vi "Alazar module.vi"(7 "FFT Channel":u32(ring)=1 items=["A"=1, "B"=2, "A + B"=3, "C"=4, "A + C"=5, "A + B"=6, "D"=8, "A + D"=9, "B + D"=10, "C + D"=12, "A + B + C + D"=15], 8 "Error in":errorcluster, 10 "Scan Status in":T1) -> (0 "Error Out":errorcluster, 3 "FFT Buffer":sgl[](array[numeric]))   [LabVIEW 2018]
uses:
  Controls/scan status.ctl
  Hardware Mfg/AlazarTech SDK/Controls/Alazar Engine Actions.ctl
  Controls/FGV Actions.ctl
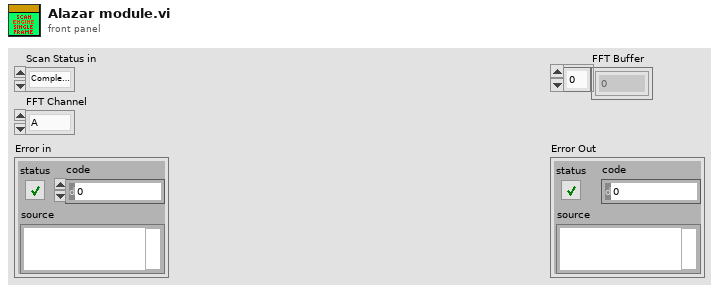
[diagram p1: front panel]
types:
  T1 = typedef "scan status.ctl" = enum16{"Complete Scan", "Start", "Continue Scan", "Finish Scan"}
  T2 = typedef "Alazar Engine Actions.ctl" = enum16{"Init", "Config Clock", "Config Ch", "Config Trig", "Config Non-FFT Acq.", "Non-FFT Acquire", "start acquire", "Config Acq.", "Acquire", "UnInit"}
  T3 = typedef "FGV Actions.ctl" = enum16{"Init", "Set", "Get", "Clear"}
  T4 = enum16{"Configure channels", "Write Scan Pattern", "Start Galvo Task", "Is Task Done?", "Stop Galvo", "Uninit", "Init: Calc scan pattern"}
  T5 = typedef "System Parameters.ctl" = cluster{"Optical Parameters":T6, "Vibratome":T7, "Table Stages":T8, "Imaging Parameter":T11, "Galvo HW Parameters":cluster{"Analog Out Channel":tag, "Min Voltage":dbl, "Max Voltage":dbl, "Pixel Clock Source":tag, "Sample Rate":dbl, "Line Clock Out Ch":tag}, "Alazar parameters":T13, "Mosaic Paramter":cluster{"X Axis":cluster{"Start [mm]":dbl, "Steps [pts]":u16, "End [mm]":dbl}, "Y Axis":cluster{"Start [mm]":dbl, "Steps [pts]":u16, "End [mm]":dbl}, "Scan Pattern":enum16{"Uni-directional", "Bi-Directional", "Spiral Out", "Spiral In"}, "Overlap Options":cluster{"Overlap Type":enum16{"No Overlap", "X Only", "Y Only", "X and Y"}, "Percent Overlap":u8, "Justify":enum16{"Start", "Center", "End"}}}, "Vibratome Axis":cluster{"Start [mm](next cut height)":dbl, "thick[um]":dbl, "#slices":dbl}}
  T6 = typedef "Optical Parameters.ctl" = cluster{"Obj. Focal Length [mm]":dbl, "Scan Lens EFL[mm]":dbl, "Tube Lens EFL[mm]":dbl, "Galvo V Range (+/-)":dbl, "Galvo Max Half Angle [Deg]":dbl, "Max Galvo Range[%]":dbl}
  T7 = typedef "Vibratome Parameters.ctl" = cluster{"Z Bottom [mm]":dbl, "Pre Cut Dwell [s]":dbl, "Blade Frequency [RPM]":u16, "Slice Speed [mm/s]":dbl, "Post Cut Dwell [s]":dbl, "Ramp Time [s]":dbl, "Start X [mm]":dbl, "Start Y [mm]":dbl, "Slice Length [mm]":dbl, "Slice Axis":enum16{"X Axis", "Y Axis", "Z Axis"}, "Controller VISA Ref":refnum<visa-resource-name>}
  T8 = typedef "Translation Stage Parameters.ctl" = cluster{"X Stage":T9, "Y Stage":T9, "Z Stage":T9}
  T9 = typedef "Translation Stage Cluster.ctl" = cluster{"Position":dbl, "Is.Enabled?":bool, "Is.Connected?":bool, "Device SN":string, "AccelerationMaximum":dbl, "VelocityMaximum":dbl, "Acceleration":dbl, "Velocity":dbl, "waitTimeout (ms)":i32, "Model":T10, "Is.Homed?":bool}
  T10 = typedef "Translation Stage Types.ctl" = enum16{"None", "Thorlabs LTS", "Thorlabs MLJ"}
  T11 = typedef "Imaging Parameters.ctl" = cluster{"Raster Scan Direction":T12, "Pixel Dwell Time [Clock Cycles]":u16, "Flyback Time [Clock Cycles]":u16, "XY Center [um]":cluster{"X":dbl, "Y":dbl}, "Pixel Step Size [um]":dbl, "XY Image Size":enum16{"32 x 32", "64 x 64", "128 x 128", "256 x 256", "512 x 512", "1024 x 1024", "2048 x 2048"}, "Custom":bool, "Custom Size":cluster{"X":u16, "Y":u16}, "Line Averages":u8}
  T12 = typedef "Scan Direction.ctl" = enum16{"Uni Directional", "Bi Directional", "None"}
  T13 = typedef "Alazar parameters.ctl" = cluster{"Trigger Settings":cluster{"General Trigger Settings":T14, "Trigger Engine 1":T15, "Trigger Engine 2":T15}, "Capture Clock":T16, "Device ID":T17, "Ch A Input Control":T18, "Ch B Input Control":T18, "Acq Settings":T19}
  T14 = typedef "General Trigger Settings.ctl" = cluster{"Trigger Operation":u32, "Coupling ID":u32, "Range ID":u32, "Delay":u32, "Timeout Ticks":u32, "Mode":u32, "Parameter":u32}
  T15 = typedef "Trigger Engine Controls.ctl" = cluster{"Trigger Engine":u32, "Source":u32, "Slope":u32, "Level":u32}
  T16 = typedef "Clock Controls.ctl" = cluster{"Sample Rate":u32, "Decimation":u32, "Source":u32, "Edge":u32}
  T17 = typedef "Alazar Device ID.ctl" = cluster{"System ID":u32, "Board ID":u32}
  T18 = typedef "Channel Input Controls.ctl" = cluster{"Channel":u8, "Coupling":u32, "Range":u32, "Impedance":u32}
  T19 = typedef "Alazar Acquisition Settings.ctl" = cluster{"Record Length":u32, "Offset":u32, "Records Per Buffer":u32, "Records Count (Records/Acq)":u32, "Window Type":u32, "Footer":u32, "Samples per record":u32, "Output Format":u32}
  T20 = cluster{"General Trigger Settings":T14, "Trigger Engine 1":T15, "Trigger Engine 2":T15}
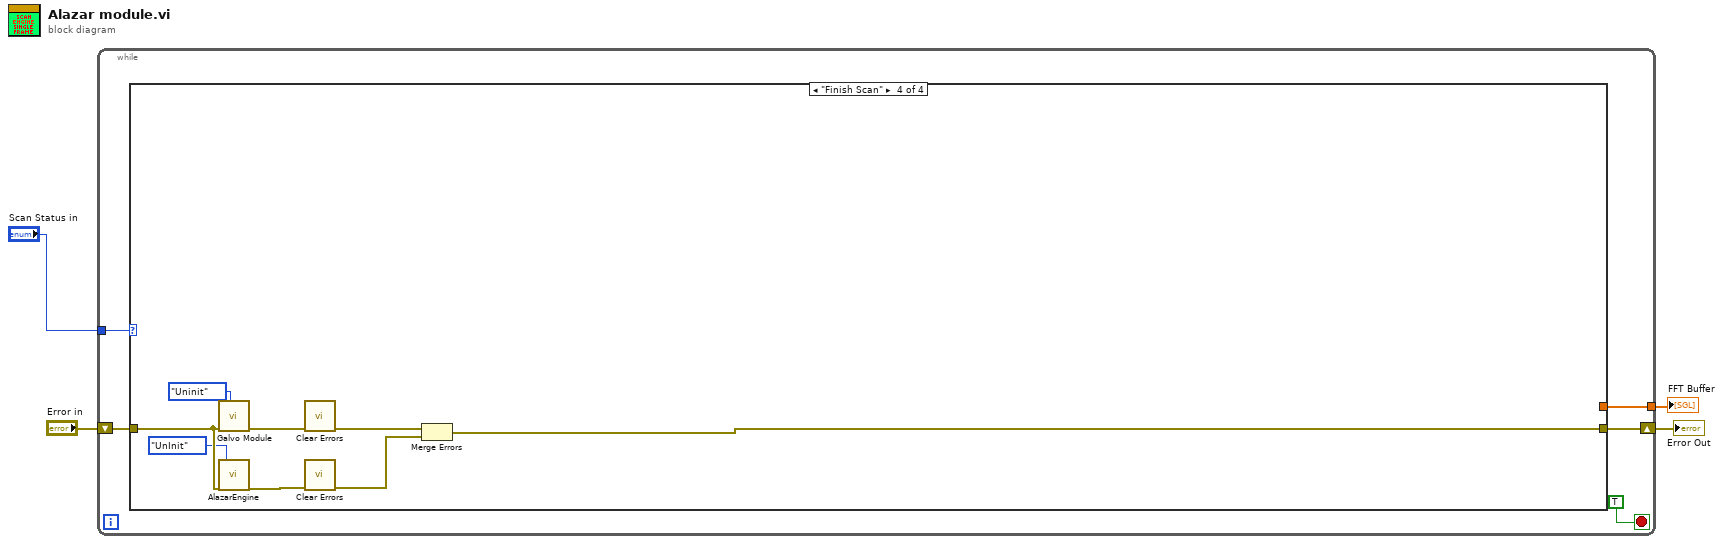
[diagram p0: block diagram]
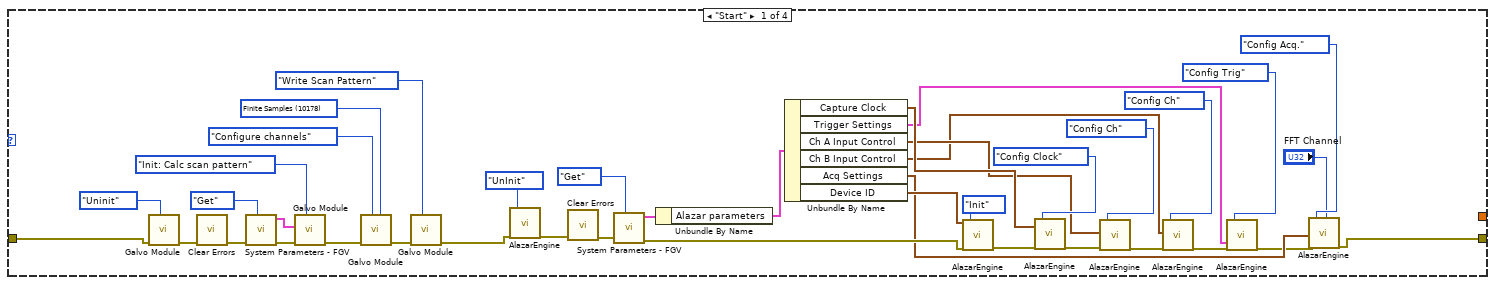
[diagram p2: hidden frame]
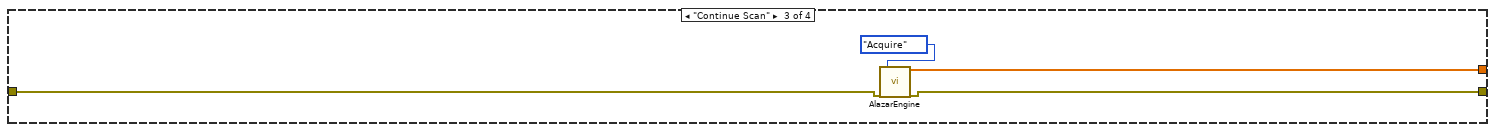
[diagram p4: hidden frame]
diagram:
  n1 = while {
    shift-right: [w8] -> w3
    shift-left: "Error in" -> [w6]
    tunnel: "Scan Status in" -> [w7]
    tunnel: [w5] -> w1
    stop <- TRUE ("Status In") stop-if-true
    n2 = case shown="\"Finish Scan\"" w7 {
      tunnel: w6 -> [w37 w50 w53 w59]
      tunnel: [w11 w50 w52 w56] -> w8
      tunnel: [_ _ w51 _] -> w5
      frame "Start" {
        w46 = 10178 items=["Finite Samples"=10178, "Continuous Samples"=10123, "Hardware Timed Single Point"=12522] ("sample mode")
        n3 = call "Galvo Module.vi"("Action"=T4."Uninit", "error in (no error)"=w37) -> ("error out"=w40:errorcluster)  [unwired: 8 in, 1 out]
        n4 = call <vilib>:"Clear Errors.vi"("error in (no error)"=w40) -> ("error out"=w38:errorcluster)  [unwired: 5 in, 1 out]
        n5 = call "System Parameters - FGV.vi"("Actions"=FGV_Actions."Get", "Error In"=w38) -> ("Error Out"=w41:errorcluster, "System Parameters"=w42:T5)  [unwired: 8 in]
        n6 = call "Galvo Module.vi"("Action"=T4."Init: Calc scan pattern", "error in (no error)"=w41, "System Parameters"=w42) -> ("error out"=w48:errorcluster)  [unwired: 7 in, 1 out]
        n7 = call "Galvo Module.vi"("sample mode"=w46, "Action"=T4."Configure channels", "error in (no error)"=w48) -> ("error out"=w49:errorcluster)  [unwired: 7 in, 1 out]
        n8 = call "Galvo Module.vi"("Action"=T4."Write Scan Pattern", "error in (no error)"=w49) -> ("error out"=w32:errorcluster)  [unwired: 8 in, 1 out]
        n9 = call "AlazarEngine.vi"("error in (no error)"=w32, "Action"=Alazar_Engine_Actions."UnInit") -> ("error out"=w31:errorcluster)  [unwired: 15 in, 2 out]
        n10 = call <vilib>:"Clear Errors.vi"("error in (no error)"=w31) -> ("error out"=w33:errorcluster)  [unwired: 5 in, 1 out]
        n11 = call "System Parameters - FGV.vi"("Actions"=FGV_Actions."Get", "Error In"=w33) -> ("Error Out"=w23:errorcluster, "System Parameters"=w35:T5)  [unwired: 8 in]
        n12 = Unbundle By Name(w35) -> ("Alazar parameters"=w34:T13)
        n13 = Unbundle By Name(w34) -> ("Capture Clock"=w21:T16, "Trigger Settings"=w18:T20, "Ch A Input Control"=w20:T18, "Ch B Input Control"=w19:T18, "Acq Settings"=w17:T19, "Device ID"=w22:T17)
        n14 = call "AlazarEngine.vi"("Device ID"=w22, "error in (no error)"=w23, "Action"=Alazar_Engine_Actions."Init") -> ("error out"=w16:errorcluster)  [unwired: 14 in, 2 out]
        n15 = call "AlazarEngine.vi"("Capture Clock"=w21, "error in (no error)"=w16, "Action"=Alazar_Engine_Actions."Config Clock") -> ("error out"=w15:errorcluster)  [unwired: 14 in, 2 out]
        n16 = call "AlazarEngine.vi"("Ch Input Control"=w20, "error in (no error)"=w15, "Action"=Alazar_Engine_Actions."Config Ch") -> ("error out"=w14:errorcluster)  [unwired: 14 in, 2 out]
        n17 = call "AlazarEngine.vi"("Ch Input Control"=w19, "error in (no error)"=w14, "Action"=Alazar_Engine_Actions."Config Ch") -> ("error out"=w13:errorcluster)  [unwired: 14 in, 2 out]
        n18 = call "AlazarEngine.vi"("Trigger Settings"=w18, "error in (no error)"=w13, "Action"=Alazar_Engine_Actions."Config Trig") -> ("error out"=w12:errorcluster)  [unwired: 14 in, 2 out]
        n19 = call "AlazarEngine.vi"("Acq Settings"=w17, "error in (no error)"=w12, "Action"=Alazar_Engine_Actions."Config Acq.", "FFT Channel"="FFT Channel") -> ("error out"=w11:errorcluster)  [unwired: 13 in, 2 out]
      }
      frame Default {
      }
      frame "Continue Scan" {
        n20 = call "AlazarEngine.vi"("error in (no error)"=w53, "Action"=Alazar_Engine_Actions."Acquire") -> ("FFT Buffer"=w51:sgl[], "error out"=w52:errorcluster)  [unwired: 15 in, 1 out]
      }
      frame "Finish Scan" {
        n21 = call "Galvo Module.vi"("Action"=T4."Uninit", "error in (no error)"=w59) -> ("error out"=w62:errorcluster)  [unwired: 8 in, 1 out]
        n22 = call "AlazarEngine.vi"("error in (no error)"=w59, "Action"=Alazar_Engine_Actions."UnInit") -> ("error out"=w61:errorcluster)  [unwired: 15 in, 2 out]
        n23 = call <vilib>:"Clear Errors.vi"("error in (no error)"=w62) -> ("error out"=w58:errorcluster)  [unwired: 5 in, 1 out]
        n24 = call <vilib>:"Clear Errors.vi"("error in (no error)"=w61) -> ("error out"=w57:errorcluster)  [unwired: 5 in, 1 out]
        n25 = Merge Errors(w58, w57) -> (w56:errorcluster)
      }
    }
  }
  "Error Out" <- w3
  "FFT Buffer" <- w1
